vi "run.create_from_asset.vi"(8 "error in":errorcluster, 11 "Nominal Client in":refnum<class "Nominal Client.lvclass">) -> (0 "error out":errorcluster, 3 "Nominal Client out":refnum<class "Nominal Client.lvclass">)   [LabVIEW 2020, in "Nominal Client.lvclass"]
uses:
  Nominal Client.lvclass
  Nominal Client.lvclass/Nominal Client.ctl
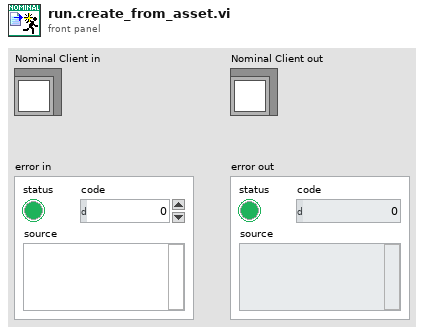
[diagram p1: front panel]
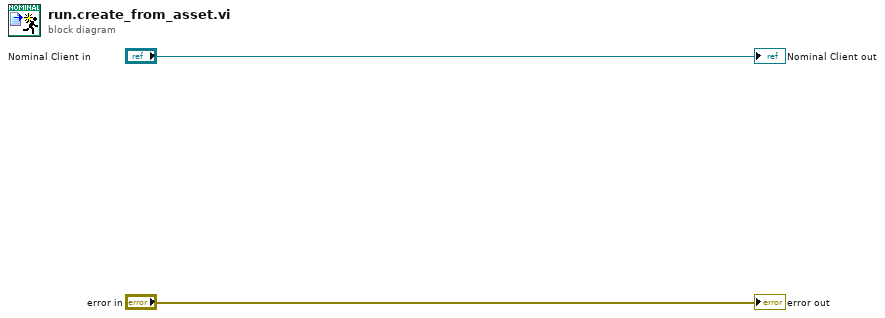
[diagram p0: block diagram]
diagram:
  "Nominal Client out" <- "Nominal Client in"
  "error out" <- "error in"
